vi "LJ Stream Config.vi"() -> ()   [LabVIEW 2020]
panel:
  out "Scans To Read":dbl=1000.0 format="%.3f"
  out "Handle Out":i32
  out "error out":errorcluster
  out "# Channels":i32
  out "Actual Scan Rate (Hz)":dbl=1000.0 format="%.3f"
  in  "AIN Range":u8(ring) items=["LJ_rgBIP10V", "LJ_rgBIP1V", "LJ_rgBIPP1V", "LJ_rgBIPP01V"]
  in  "Display Rate (Hz)":i32=1
  in  "Binary":bool
  in  "StreamSettlingFactor":i32
  in  "Resolution Index":u8
  in  "PC buffer size (seconds)":dbl=10.0 format="%.2f"
  in  "Scan Rate (Hz)":dbl=1000.0 format="%.3f"
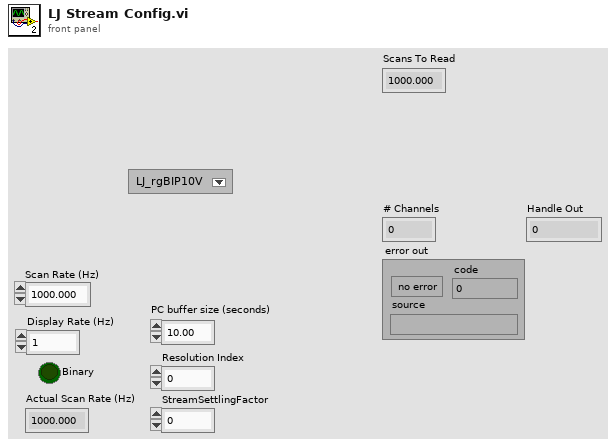
[diagram p1: front panel]
types:
  T1 = cluster{"PC buffer size (seconds)":dbl, "Resolution Index":u8, "StreamSettlingFactor":i32, "Binary":bool}
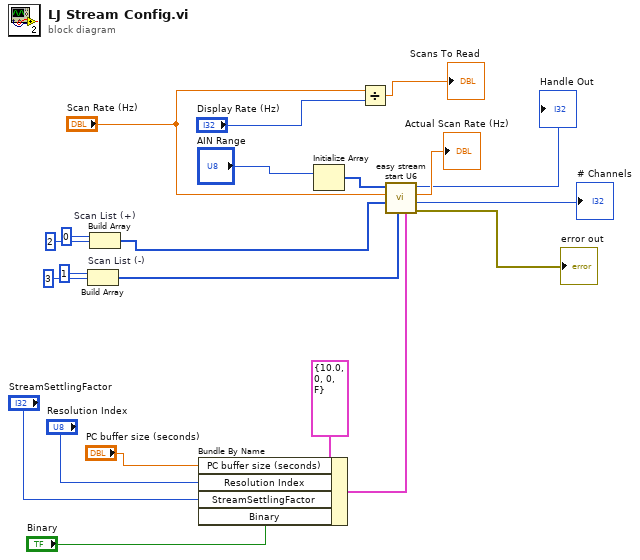
[diagram p0: block diagram]
diagram:
  n1 = Build Array "Scan List (-)"(1 ("SettlingFactor"), 3 ("SettlingFactor")) -> (w8:i32[])
  n2 = Build Array "Scan List (+)"(0 ("SettlingFactor"), 2 ("SettlingFactor")) -> (w11:i32[])
  n3 = Bundle By Name(cluster=T1 {"PC buffer size (seconds)"=10.0, "Resolution Index"=0, "StreamSettlingFactor"=0, "Binary"=FALSE} ("Advanced"), "PC buffer size (seconds)"="PC buffer size (seconds)", "Resolution Index"="Resolution Index", "StreamSettlingFactor"="StreamSettlingFactor", "Binary"="Binary") -> (w17:T1)
  n4 = Initialize Array("AIN Range") -> (w13:u8[])  [unwired: 1 in]
  n5 = Divide(x="Scan Rate (Hz)", y="Display Rate (Hz)") -> (x/y=→"Scans To Read":dbl)
  n6 = call "easy stream start U6.vi"("Advanced"=w17, "Scan List (-)"=w8, "Scan List (+)"=w11, "Scan Rate (Hz)"="Scan Rate (Hz)", "Range Constants"=w13) -> ("error out"=→"error out":errorcluster, "# Channels"=→"# Channels":i32, "Actual Scan Rate (Hz)"=→"Actual Scan Rate (Hz)":dbl, "Handle Out"=→"Handle Out":i32)  [unwired: 3 in]
